vi "Generate Concrete Relative Paths File.vi"() -> ()   [LabVIEW 2023]
uses:
  Abstract Class/Abstract Class.lvclass
  Concrete Classes/Class 1/Class 1.lvclass
  C:/Projects/Class Loader/Tests/Abstract Class/Abstract Class.lvclass
  Concrete Classes/Class 2/Class 2.lvclass
  Concrete Classes/Class 3/Class 3 Folder/Class 3.lvclass
  Concrete Classes/Class 4/Class 4.lvclass
  Concrete Classes/Class 5/Class 5.lvclass
  Concrete Classes/Class 6/Class 6.lvclass
  Concrete Classes/Class 7/Class 7.lvclass
  Concrete Classes/Class 8/Class 8.lvclass
  Concrete Classes/Class 9/Class 9.lvclass
  Concrete Classes/Class 10/Class 10.lvclass
  C:/Projects/Class Loader/Tests/Concrete Classes/Class 1/Class 1.lvclass
  C:/Projects/Class Loader/Tests/Concrete Classes/Class 2/Class 2.lvclass
  C:/Projects/Class Loader/Tests/Concrete Classes/Class 3/Class 3 Folder/Class 3.lvclass
  C:/Projects/Class Loader/Tests/Concrete Classes/Class 4/Class 4.lvclass
  C:/Projects/Class Loader/Tests/Concrete Classes/Class 5/Class 5.lvclass
  C:/Projects/Class Loader/Tests/Concrete Classes/Class 6/Class 6.lvclass
  C:/Projects/Class Loader/Tests/Concrete Classes/Class 7/Class 7.lvclass
  C:/Projects/Class Loader/Tests/Concrete Classes/Class 8/Class 8.lvclass
  C:/Projects/Class Loader/Tests/Concrete Classes/Class 9/Class 9.lvclass
  C:/Projects/Class Loader/Tests/Concrete Classes/Class 10/Class 10.lvclass
  Class Loader/Class Loader/Class Loader.lvclass
panel:
  out "error out":errorcluster
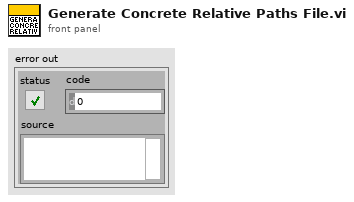
[diagram p1: front panel]
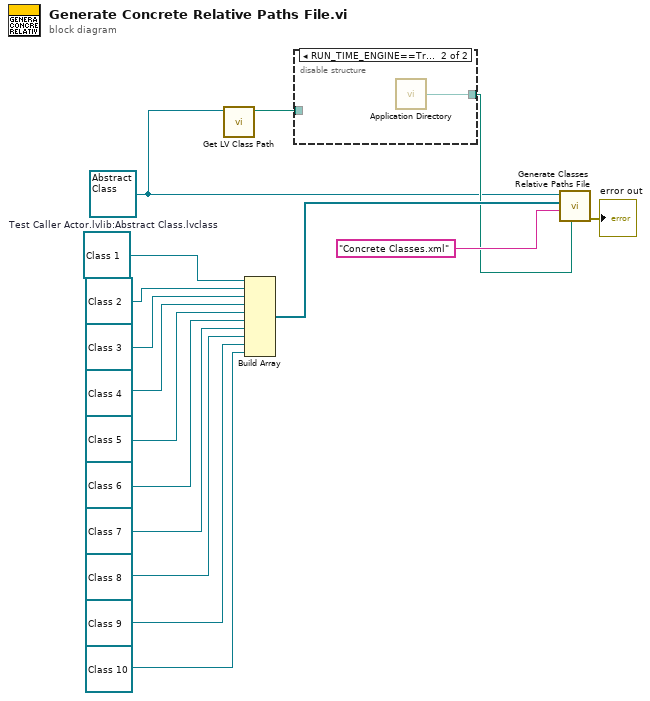
[diagram p0: block diagram]
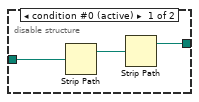
[diagram p2: hidden frame]
diagram:
  w1 = refnum<class "Abstract Class.lvclass"> refnum  # Test Caller Actor.lvlib:Abstract Class.lvclass
  n1 = call <vilib>:"Get LV Class Path.vi"("object"=w1) -> ("class path"=w3:path)  [unwired: 9 in, 1 out]
  n2 = Build Array(refnum<class "Class 1.lvclass"> refnum ("Concrete Classes.lvlib:Class 1.lvclass"), refnum<class "Class 2.lvclass"> refnum ("Concrete Classes.lvlib:Class 2.lvclass"), refnum<class "Class 3.lvclass"> refnum ("Concrete Classes.lvlib:Class 3.lvclass"), refnum<class "Class 4.lvclass"> refnum ("Concrete Classes.lvlib:Class 4.lvclass"), refnum<class "Class 5.lvclass"> refnum ("Concrete Classes.lvlib:Class 5.lvclass"), refnum<class "Class 6.lvclass"> refnum ("Concrete Classes.lvlib:Class 6.lvclass"), refnum<class "Class 7.lvclass"> refnum ("Concrete Classes.lvlib:Class 7.lvclass"), refnum<class "Class 8.lvclass"> refnum ("Concrete Classes.lvlib:Class 8.lvclass"), refnum<class "Class 9.lvclass"> refnum ("Concrete Classes.lvlib:Class 9.lvclass"), refnum<class "Class 10.lvclass"> refnum ("Concrete Classes.lvlib:Class 10.lvclass")) -> (w7:refnum<class "Abstract Class.lvclass">[])
  n3 = disable-structure shown="RUN_TIME_ENGINE==True" {
    disable-tunnel: [w18 w20] -> w2
    disable-tunnel: w3 -> [w17 _]
    frame condition #0 (active) {
      n4 = Strip Path(path=w17) -> (stripped path=w19:path)  [unwired: 1 out]
      n5 = Strip Path(path=w19) -> (stripped path=w18:path)  [unwired: 1 out]
    }
    frame condition #1 {
      n6 = call <vilib>:"Application Directory.vi"() -> ("Application Directory"=w20:path)
    }
  }
  n7 = call "Generate Classes Relative Paths File.vi"("Relative Paths File Path"=w2, "Relative Paths File Name"="Concrete Classes.xml", "Classes"=w7, "Reference Class"=w1) -> ("error out"=→"error out":errorcluster)  [unwired: 7 in]
